vi "Peregrine_move_with_status.vi"(0 "Handle in":refnum<visa-resource-name>, 2 "Address":u8, 5 "Target":i32, 7 "Speed":i16, 9 "Acceleration":u16, 11 "error":errorcluster) -> (4 "Handle out":refnum<visa-resource-name>, 6 "Speed\nresponse":i16, 8 "Position\nresponse":i32, 13 "Flags\nmoveS":T1, 15 "error out":errorcluster)   [LabVIEW 2019]
panel:
  in  "Flags bundle":T1
  out "Command\nresponse":i32
  out "Address response":u8
  # "Inputs"
  # "Response message"
  # "Output"
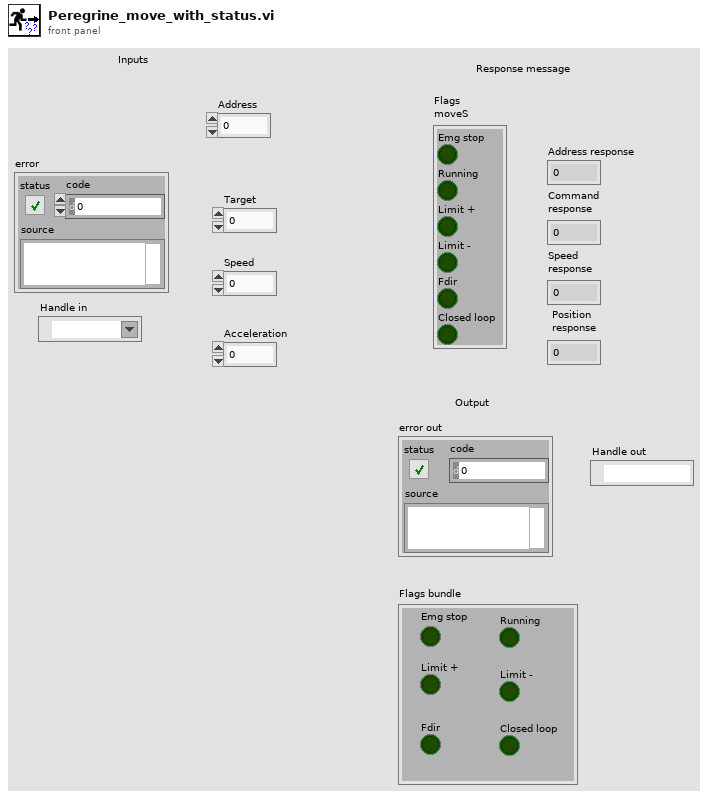
[diagram p1: front panel]
types:
  T1 = cluster{"Emg stop":bool, "Running":bool, "Limit +":bool, "Limit -":bool, "Fdir":bool, "Closed loop":bool}
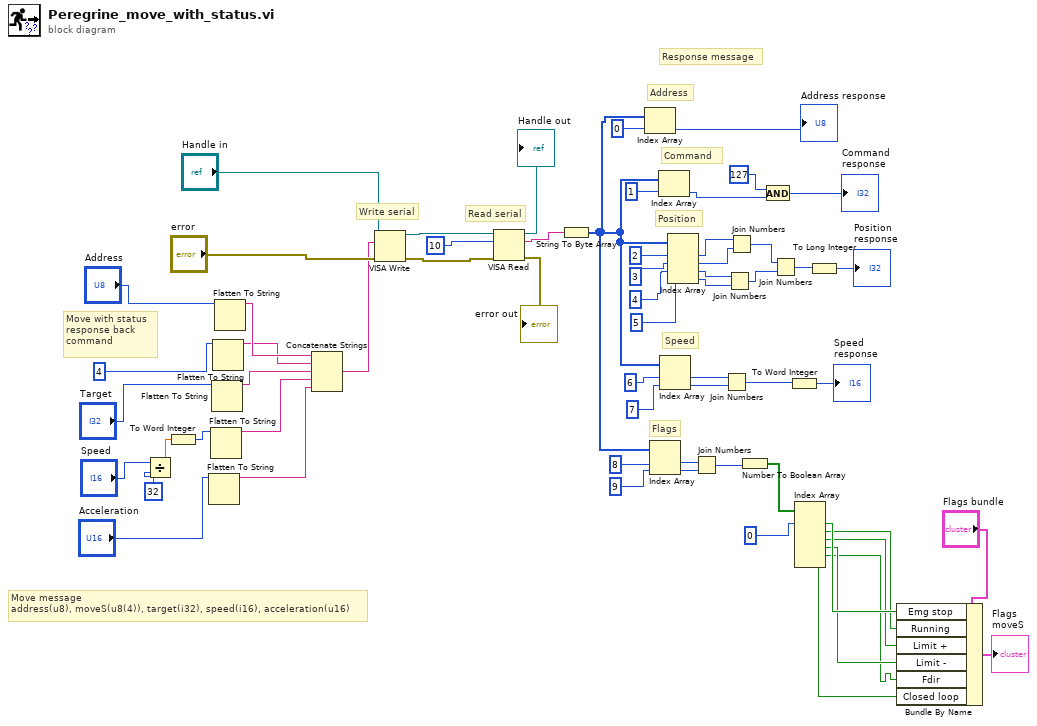
[diagram p0: block diagram]
diagram:
  # "Response message"
  # "Move with status\nresponse back\ncommand"
  # "Command"
  # "Address"
  # "Flags"
  # "Speed"
  # "Position"
  # "Read serial"
  # "Write serial"
  # "Move message\naddress(u8), moveS(u8(4)), target(i32), speed(i16), acceleration(u16)"
  n1 = Divide(x="Speed", y=32) -> (x/y=w2:dbl)
  n2 = To Word Integer(number=w2) -> (16bit integer=w1:i16)
  n3 = Flatten To String(anything="Acceleration") -> (data string=w6:string)  [unwired: 3 in, 2 out]
  n4 = Flatten To String(anything=w1) -> (data string=w7:string)  [unwired: 3 in, 2 out]
  n5 = Flatten To String(anything="Target") -> (data string=w8:string)  [unwired: 3 in, 2 out]
  n6 = Flatten To String(anything=u8 4) -> (data string=w9:string)  [unwired: 3 in, 2 out]
  n7 = Flatten To String(anything="Address") -> (data string=w13:string)  [unwired: 3 in, 2 out]
  n8 = Concatenate Strings(w13, w9, w8, w7, w6) -> (w5:string)
  n9 = VISA Write(VISA resource name="Handle in", write buffer=w5, error in (no error)="error") -> (VISA resource name out=w62:refnum<visa-resource-name>, error out=w23:errorcluster)  [unwired: 1 out]
  n10 = VISA Read(VISA resource name=w62, byte count=10, error in (no error)=w23) -> (VISA resource name out=→"Handle out":refnum<visa-resource-name>, read buffer=w60:string, error out=→"error out":errorcluster)  [unwired: 1 out]
  n11 = String To Byte Array(string=w60) -> (unsigned byte array=w52:u8[])
  n12 = Index Array(array=w52, index=0) -> (element=→"Address response":u8)
  n13 = Index Array(array=w52, index #1=8, index #2=9) -> (element #1=w42:u8, element #2=w41:u8)
  n14 = Index Array(array=w52, index=1) -> (element=w44:u8)
  n15 = Index Array(array=w52, index #1=6, index #2=7) -> (element #1=w34:u8, element #2=w33:u8)
  n16 = Index Array(array=w52, index #1=2, index #2=3, index #3=4, index #4=5) -> (element #1=w50:u8, element #2=w49:u8, element #3=w48:u8, element #4=w47:u8)
  n17 = Join Numbers(hi=w42, lo=w41) -> ((hi.lo)=w39:u16)
  n18 = Join Numbers(hi=w34, lo=w33) -> ((hi.lo)=w32:u16)
  n19 = Join Numbers(hi=w48, lo=w47) -> ((hi.lo)=w46:u16)
  n20 = Join Numbers(hi=w50, lo=w49) -> ((hi.lo)=w45:u16)
  n21 = Number To Boolean Array(number=w39) -> (Boolean array=w37:bool[])
  n22 = And(x=127, y=w44) -> (x .and. y?=→"Command\nresponse":i32)
  n23 = Join Numbers(hi=w45, lo=w46) -> ((hi.lo)=w40:u32)
  n24 = To Word Integer(number=w32) -> (16bit integer=→"Speed\nresponse":i16)
  n25 = Index Array(array=w37, index #1=0) -> (element #1=w21:bool, element #2=w20:bool, element #3=w19:bool, element #4=w18:bool, element #5=w17:bool, element #6=w16:bool)  [unwired: 5 in]
  n26 = To Long Integer(number=w40) -> (32bit integer=→"Position\nresponse":i32)
  n27 = Bundle By Name(cluster="Flags bundle", "Emg stop"=w21, "Running"=w20, "Limit +"=w19, "Limit -"=w18, "Fdir"=w17, "Closed loop"=w16) -> (→"Flags\nmoveS":T1)
